vi "from string.vi"(8 "error in":errorcluster, 9 "data":string, 10 "version":string, 11 "fixed channel configuration in":refnum<class "WaveformAcq configuration.lvclass">) -> (0 "error out":errorcluster, 3 "fixed channel configuration out":refnum<class "WaveformAcq configuration.lvclass">)   [LabVIEW 2017, in "WaveformAcq configuration.lvclass"]
doc: "Provides an interface for loading a module configuration from a file or other serialized data source. It is recommended that all children of this class store data in two sets--data required for its own initialization, and any data required for parent initialization--and that each implementation uses the <b>Call Parent Method</b> primitive to de-serialize parent information. As a result, it is expected that every module configuration class calls <b>component configuration.lvclass:From String.vi</b>.\nNI Tag Bus Module Framework 1.0.3.43\nNI Systems Engineering"
uses:
  WaveformAcq configuration.lvclass
  WaveformAcq configuration.lvclass/WaveformAcq configuration.ctl
  <vilib>/NI/DCAF/Tag Editor Core/control module/configuration/control module configuration.lvclass
  <vilib>/NI/Configuration Framework/serializable configuration/NISE_CEF_serializable configuration.lvclass
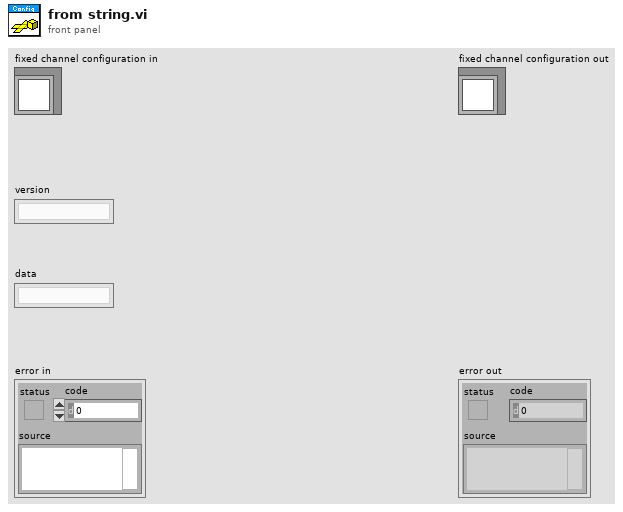
[diagram p1: front panel]
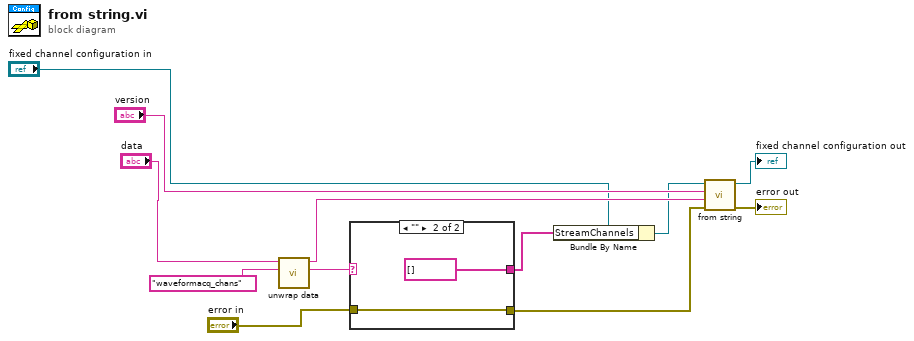
[diagram p0: block diagram]
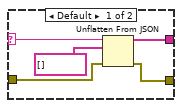
[diagram p2: hidden frame]
diagram:
  n1 = call <vilib>:"unwrap data.vi"("identifier"="waveformacq_chans", "data to unwrap"="data") -> ("unwrapped data"=w6:string, "remaining string"=w7:string)  [unwired: 8 in]
  n2 = case shown="\"\"" w6 {
    selector: w6 -> [w17 _]
    tunnel: [w16 string[] []] -> w3
    tunnel: "error in" -> [w14 w18]
    tunnel: [w13 w18] -> w4
    frame Default {
      n3 = Unflatten From JSON(JSON string=w17, type and defaults=string[] [], error in (no error)=w14) -> (value=w16:string[], error out=w13:errorcluster)  [unwired: 4 in]
    }
    frame "" {
    }
  }
  n4 = Bundle By Name(cluster="fixed channel configuration in", "StreamChannels"=w3) -> (w1:refnum<class "WaveformAcq configuration.lvclass">)
  n5 = call-parent "from string.vi"("error in"=w4, "data"=w7, "version"="version", "fixed channel configuration in"=w1) -> ("error out"=→"error out":errorcluster, "fixed channel configuration out"=→"fixed channel configuration out":refnum<class "WaveformAcq configuration.lvclass">)  [unwired: 6 in]
